vi "Software close.vi"(8 "error in":errorcluster) -> (0 "error out":errorcluster)   [LabVIEW 2019]
doc: "Close all notifiers and user events references.\n\n------------------\nJuan Navarro\nLab It Studio"
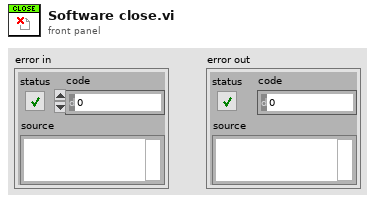
[diagram p1: front panel]
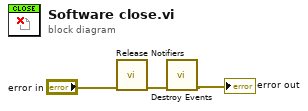
[diagram p0: block diagram]
diagram:
  n1 = call "Release Notifiers.vi"("error in"="error in") -> ("error out"=w2:errorcluster)  [unwired: 10 in]
  n2 = call "Destroy Events.vi"("error in"=w2) -> ("error out"=→"error out":errorcluster)  [unwired: 10 in]
